vi "gMODE.vi"() -> ()   [LabVIEW 2011]
panel:
  out "gMODE":bool
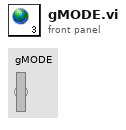
[diagram p1: front panel]
diagram:
